vi "Number of Images in Current Set FGV.vi"(7 "Operation":enum16{"GET", "SET"}(ring), 8 "Error In":errorcluster, 11 "Number of pics taken":i32) -> (0 "Error Out":errorcluster, 3 "Number of pics taken Out":i32)   [LabVIEW 2014]
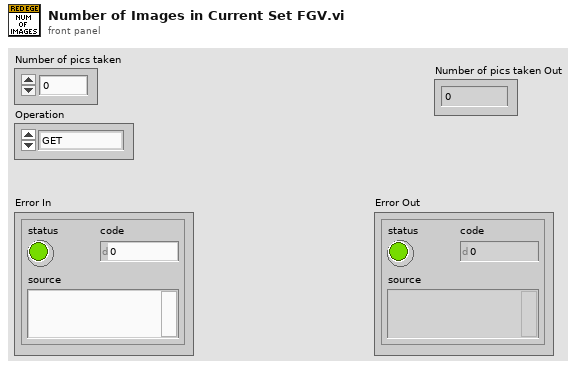
[diagram p1: front panel]
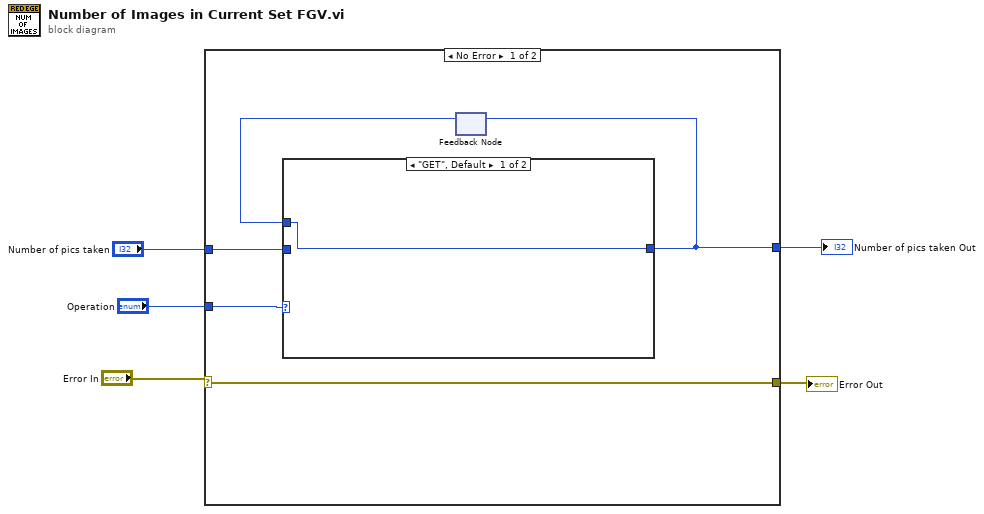
[diagram p0: block diagram]
diagram:
  n1 = case shown="No Error" "Error In" {
    selector: "Error In" -> [w6 w13]
    tunnel: "Number of pics taken" -> [w10 w14]
    tunnel: "Operation" -> [w8 _]
    tunnel: [w7 w14] -> w2
    tunnel: [w6 w13] -> w1
    frame No Error {
      n2 = feedback #1() -> (w9:i32)  [unwired: 1 in]
      n3 = case shown="\"GET\", Default" w8 {
        tunnel: [w11 w12] -> w7
        tunnel: w10 -> [_ w12]
        tunnel: w9 -> [w11 _]
        frame "GET", Default {
        }
        frame "SET" {
        }
      }
      n4 = feedback-in #1(w7) -> ()
    }
    frame Error {
    }
  }
  "Error Out" <- w1
  "Number of pics taken Out" <- w2
